vi "Update Calibration.vi"(8 "error in":errorcluster, 11 "Config in":refnum<class "Config.lvclass">) -> (0 "error out":errorcluster, 3 "Config out":refnum<class "Config.lvclass">)   [LabVIEW 2023, in "Config.lvlib" / "Config.lvclass"]
uses:
  Config.lvclass
panel:
  in  "No Cal Required":bool
  in  "OK Button":bool
  in  "Calibration Due:":timestamp
  # "Use the control below to set the calibration due date\nfor the instrument, or select No Calibration Required."
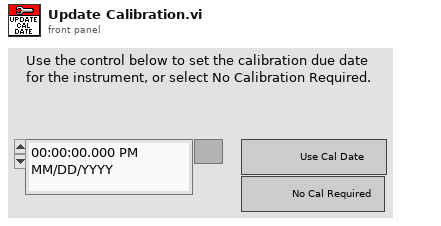
[diagram p1: front panel]
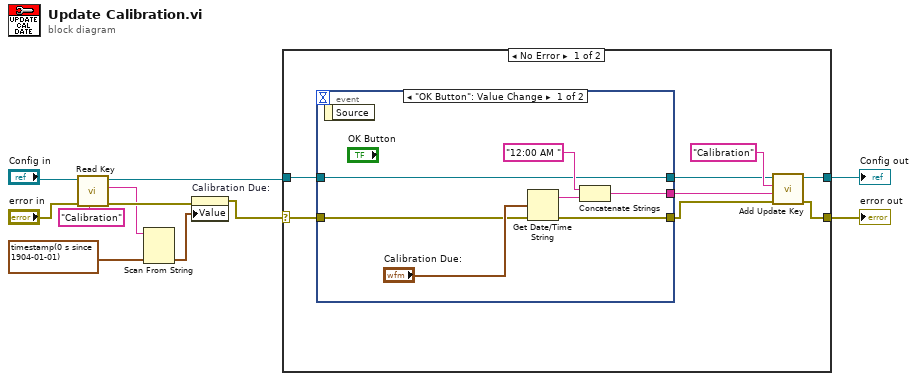
[diagram p0: block diagram]
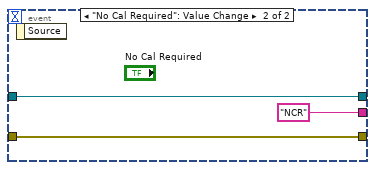
[diagram p2: hidden frame]
diagram:
  n1 = call "Read Key.vi"("Key Name"="Calibration", "error in"="error in", "Config in"="Config in") -> ("error out"=w5:errorcluster, "Key Value"=w3:string, "Config out"=w8:refnum<class "Config.lvclass">)  [unwired: 6 in]
  n2 = Scan From String(input string=w3, default 1=timestamp(0 s since 1904-01-01)) -> (output 1=w1:timestamp)  [unwired: 3 in, 3 out]
  n3 = property on="Calibration Due:" class="AbsTime (strict)"(error in=w5, "Value"=w1) -> (error out=w6:errorcluster)  [unwired: 1 in, 1 out]
  n4 = case shown="No Error" w6 {
    selector: w6 -> [w12 w29]
    tunnel: [w19 w30] -> w11
    tunnel: w8 -> [w15 w30]
    tunnel: [w13 w29] -> w10
    frame No Error {
      n5 = event shown="[0] \"OK Button\": Value Change" {
        selector: _ -> [_ _]
        dyn-events: _ -> [_ _]
        timeout: _ -> [_ _]
        tunnel: [w22 "NCR" ("Key")] -> w17
        tunnel: [w21 w28] -> w16
        tunnel: w15 -> [w21 w28]
        tunnel: [w20 w26] -> w14
        tunnel: w12 -> [w20 w26]
        event "OK Button": Value Change {
          n6 = event-data() -> ()  [unwired: 1 in, 1 out]
          n7 = Get Date/Time String(seconds (now)="Calibration Due:") -> (date string=w23:string)  [unwired: 2 in, 1 out]
          n8 = Concatenate Strings("12:00 AM ", w23) -> (w22:string)
        }
        event "No Cal Required": Value Change {
          n9 = event-data() -> ()  [unwired: 1 in, 1 out]
        }
      }
      n10 = call "Add Update Key.vi"("error in"=w14, "Value"=w17, "Key"="Calibration", "Config in"=w16) -> ("error out"=w13:errorcluster, "Config out"=w19:refnum<class "Config.lvclass">)  [unwired: 6 in]
    }
    frame Error {
    }
  }
  "error out" <- w10
  "Config out" <- w11
